vi "单独启动模块流程.vi"(11 "模块选择":T1) -> ()   [LabVIEW 2016]
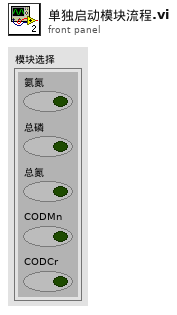
[diagram p1: front panel]
types:
  T1 = cluster{"氨氮":bool, "总磷":bool, "总氮":bool, "CODMn":bool, "CODCr":bool}
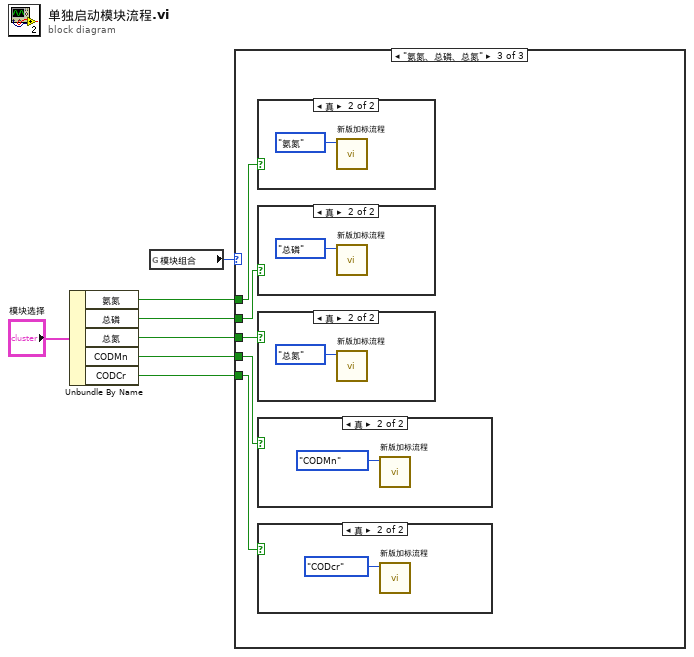
[diagram p0: block diagram]
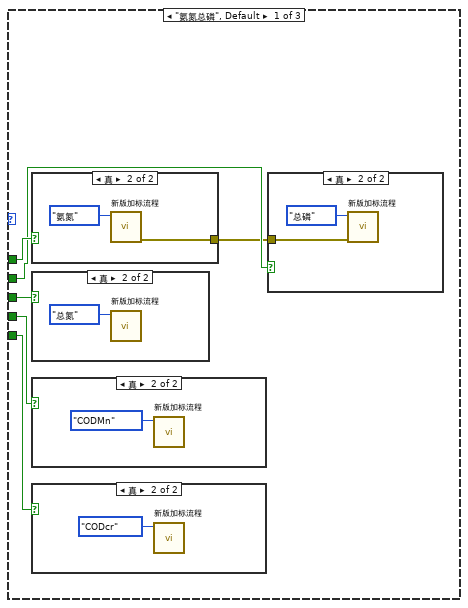
[diagram p2: hidden frame]
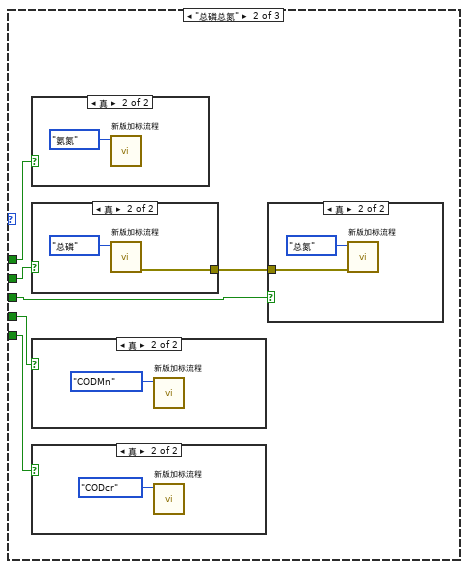
[diagram p8: hidden frame]
diagram:
  n1 = Unbundle By Name("模块选择") -> ("氨氮"=w5:bool, "总磷"=w4:bool, "总氮"=w1:bool, "CODMn"=w3:bool, "CODCr"=w2:bool)
  n2 = global read "断电保存全局.vi" "模块组合"() -> (w6:enum16{"氨氮总磷", "总磷总氮", "氨氮、总磷、总氮"})
  n3 = case shown="\"氨氮、总磷、总氮\"" w6 {
    tunnel: w5 -> [w11 w24 w36]
    tunnel: w4 -> [w10 w23 w35]
    tunnel: w3 -> [w13 w26 w38]
    tunnel: w2 -> [w12 w25 w37]
    tunnel: w1 -> [w8 w22 w34]
    frame "氨氮总磷", Default {
      n4 = case shown="真" w11 {
        tunnel: [_ w17] -> w9
        frame False {
        }
        frame True {
          n5 = call "新版加标流程.vi"("参数"=enum16{"氨氮", "总磷", "总氮", "CODMn", "CODcr"}."氨氮") -> ("error out"=w17:errorcluster)  [unwired: 10 in]
        }
      }
      n6 = case shown="真" w8 {
        frame False {
        }
        frame True {
          n7 = call "新版加标流程.vi"("参数"=enum16{"氨氮", "总磷", "总氮", "CODMn", "CODcr"}."总氮") -> ()  [unwired: 10 in, 1 out]
        }
      }
      n8 = case shown="真" w13 {
        frame False {
        }
        frame True {
          n9 = call "新版加标流程.vi"("参数"=enum16{"氨氮", "总磷", "总氮", "CODMn", "CODcr"}."CODMn") -> ()  [unwired: 10 in, 1 out]
        }
      }
      n10 = case shown="真" w12 {
        frame False {
        }
        frame True {
          n11 = call "新版加标流程.vi"("参数"=enum16{"氨氮", "总磷", "总氮", "CODMn", "CODcr"}."CODcr") -> ()  [unwired: 10 in, 1 out]
        }
      }
      n12 = case shown="真" w10 {
        tunnel: w9 -> [_ w15]
        frame False {
        }
        frame True {
          n13 = call "新版加标流程.vi"("error in (no error)"=w15, "参数"=enum16{"氨氮", "总磷", "总氮", "CODMn", "CODcr"}."总磷") -> ()  [unwired: 9 in, 1 out]
        }
      }
    }
    frame "总磷总氮" {
      n14 = case shown="真" w24 {
        frame False {
        }
        frame True {
          n15 = call "新版加标流程.vi"("参数"=enum16{"氨氮", "总磷", "总氮", "CODMn", "CODcr"}."氨氮") -> ()  [unwired: 10 in, 1 out]
        }
      }
      n16 = case shown="真" w23 {
        tunnel: [_ w29] -> w21
        frame False {
        }
        frame True {
          n17 = call "新版加标流程.vi"("参数"=enum16{"氨氮", "总磷", "总氮", "CODMn", "CODcr"}."总磷") -> ("error out"=w29:errorcluster)  [unwired: 10 in]
        }
      }
      n18 = case shown="真" w26 {
        frame False {
        }
        frame True {
          n19 = call "新版加标流程.vi"("参数"=enum16{"氨氮", "总磷", "总氮", "CODMn", "CODcr"}."CODMn") -> ()  [unwired: 10 in, 1 out]
        }
      }
      n20 = case shown="真" w25 {
        frame False {
        }
        frame True {
          n21 = call "新版加标流程.vi"("参数"=enum16{"氨氮", "总磷", "总氮", "CODMn", "CODcr"}."CODcr") -> ()  [unwired: 10 in, 1 out]
        }
      }
      n22 = case shown="真" w22 {
        tunnel: w21 -> [_ w27]
        frame False {
        }
        frame True {
          n23 = call "新版加标流程.vi"("error in (no error)"=w27, "参数"=enum16{"氨氮", "总磷", "总氮", "CODMn", "CODcr"}."总氮") -> ()  [unwired: 9 in, 1 out]
        }
      }
    }
    frame "氨氮、总磷、总氮" {
      n24 = case shown="真" w36 {
        frame False {
        }
        frame True {
          n25 = call "新版加标流程.vi"("参数"=enum16{"氨氮", "总磷", "总氮", "CODMn", "CODcr"}."氨氮") -> ()  [unwired: 10 in, 1 out]
        }
      }
      n26 = case shown="真" w35 {
        frame False {
        }
        frame True {
          n27 = call "新版加标流程.vi"("参数"=enum16{"氨氮", "总磷", "总氮", "CODMn", "CODcr"}."总磷") -> ()  [unwired: 10 in, 1 out]
        }
      }
      n28 = case shown="真" w34 {
        frame False {
        }
        frame True {
          n29 = call "新版加标流程.vi"("参数"=enum16{"氨氮", "总磷", "总氮", "CODMn", "CODcr"}."总氮") -> ()  [unwired: 10 in, 1 out]
        }
      }
      n30 = case shown="真" w38 {
        frame False {
        }
        frame True {
          n31 = call "新版加标流程.vi"("参数"=enum16{"氨氮", "总磷", "总氮", "CODMn", "CODcr"}."CODMn") -> ()  [unwired: 10 in, 1 out]
        }
      }
      n32 = case shown="真" w37 {
        frame False {
        }
        frame True {
          n33 = call "新版加标流程.vi"("参数"=enum16{"氨氮", "总磷", "总氮", "CODMn", "CODcr"}."CODcr") -> ()  [unwired: 10 in, 1 out]
        }
      }
    }
  }
